vi "SS Kill Dynamic VIs.vi"(8 "error in (no error)":errorcluster, 11 "Subsystem Class in":refnum<class "Subsystem Class.lvclass">) -> (0 "error out":errorcluster, 3 "Subsystem Class out":refnum<class "Subsystem Class.lvclass">)   [LabVIEW 2021, in "Subsystem Class.lvclass"]
uses:
  Subsystem Class.lvclass
  Subsystem Class.lvclass/Subsystem Class.ctl
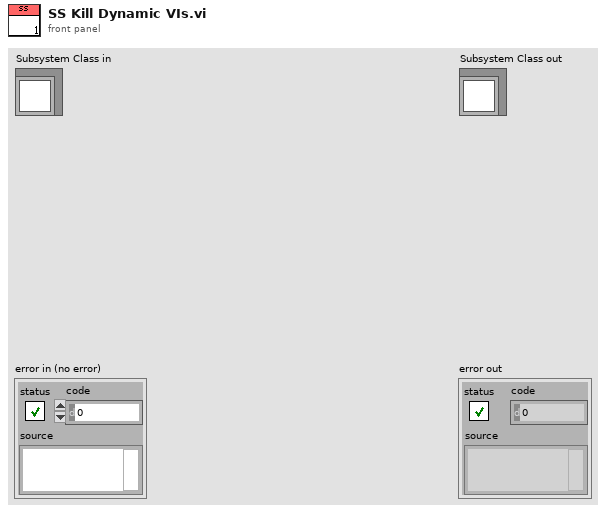
[diagram p1: front panel]
types:
  T1 = enum32{"Bad", "Idle", "Run top level", "Running"}
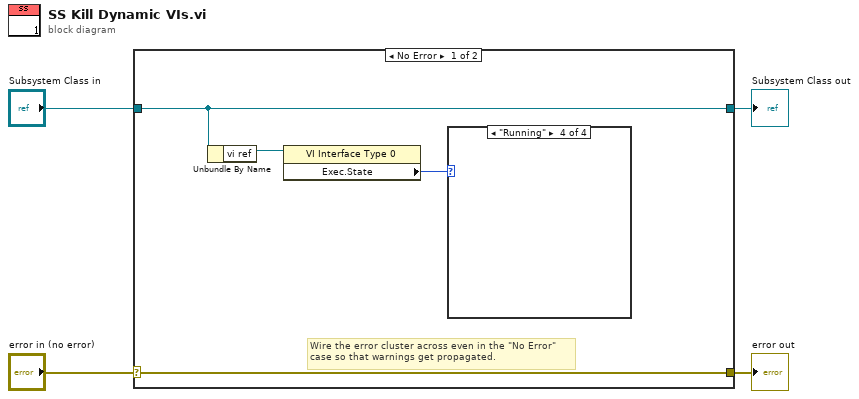
[diagram p0: block diagram]
diagram:
  n1 = case shown="No Error" "error in (no error)" {
    selector: "error in (no error)" -> [w8 w10]
    tunnel: [w8 w10] -> w3
    tunnel: [w7 w9] -> w1
    tunnel: "Subsystem Class in" -> [w7 w9]
    frame No Error {
      # "Wire the error cluster across even in the \"No Error\"\ncase so that warnings get propagated."
      n2 = Unbundle By Name(w7) -> ("vi ref"=w6:refnum<vi>)
      n3 = property class="VI Interface Type 0"(reference=w6) -> ("Exec.State"=w5:T1)  [unwired: 1 in, 2 out]
      n4 = case shown="\"Running\"" w5 {
        frame "Bad", Default {
        }
        frame "Idle" {
        }
        frame "Run top level" {
        }
        frame "Running" {
        }
      }
    }
    frame Error {
    }
  }
  "error out" <- w3
  "Subsystem Class out" <- w1
